vi "Substring.vi"() -> ()   [LabVIEW 2012]
panel:
  in  "length (rest)":i32=15
  in  "offset (0)":i32=2
  out "substring":string
  in  "String":string="Ho sceso, dandoti il braccio, almeno un milione di scale.\nE ora che non ci sei  il vuoto ad ogni gradino.\nAnche cos  stato breve il nostro lungo viaggio.\nIl mio dura tuttora, n pi mi occorrono.\nLe coincidenze, le prenotazioni,\nle trappole, gli scorni di chi crede che la realt sia quella che si vede.\n\nHo sceso milioni di scale dandoti il braccio.\nNon gi perch con quattr'occhi forse si vede di pi.\nCon te le ho scese perch sapevo che di noi due.\nLe sole vere pupille, sebbene tanto offuscate,\nerano le tue."
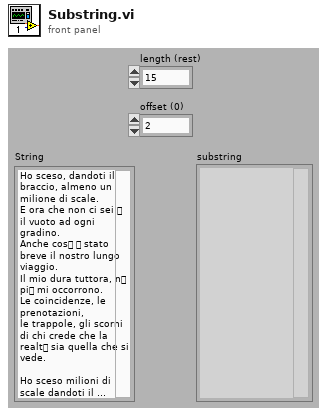
[diagram p1: front panel]
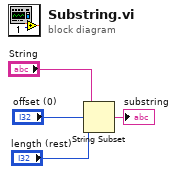
[diagram p0: block diagram]
diagram:
  n1 = String Subset(string="String", offset (0)="offset (0)", length (rest)="length (rest)") -> (substring=→"substring":string)
